vi "TIFFY Cb Crto RGB.vi"(0 "para0":cluster{}, 1 "para4":cluster{}, 2 "para6":cluster{}, 5 "para1":cluster{}, 7 "para2":cluster{}, 9 "para3":cluster{}, 11 "error in (no error)":errorcluster, 12 "para5":cluster{}) -> (3 "para4 out":cluster{}, 4 "para0 out":cluster{}, 6 "para6 out":cluster{}, 8 "function return":u32, 14 "para5 out":cluster{}, 15 "error out":errorcluster)   [LabVIEW 2018]
doc: "LIBTIFF_DLL_IMPEXP void TIFFYCbCrtoRGB(TIFFYCbCrToRGB *, uint32, int32, int32,\n uint32 *, uint32 *, uint32 *);\nextern void TIFFYCbCrtoRGB(TIFFYCbCrToRGB *, uint32, int32, int32,\n uint32 *, uint32 *, uint32 *);"
uses:
  libtiff3.dll
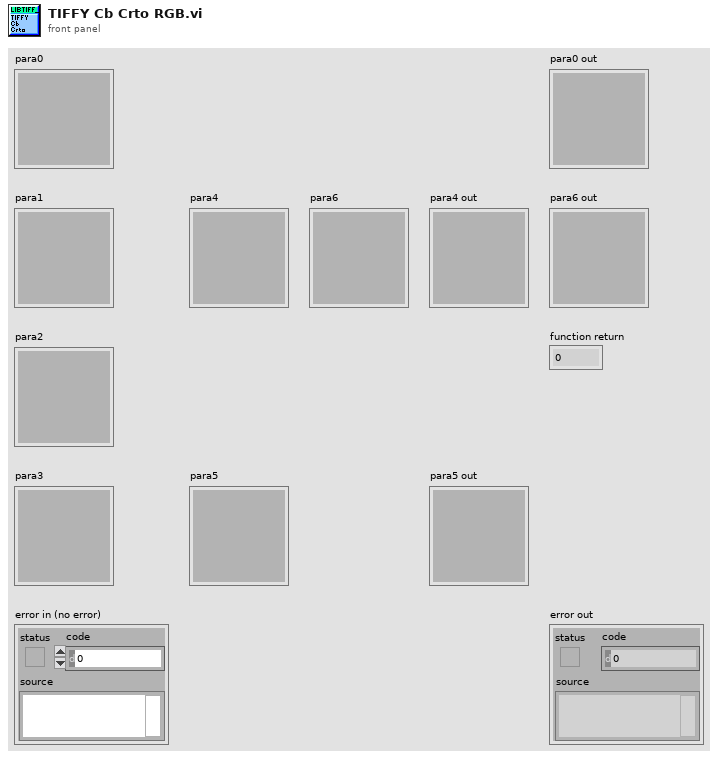
[diagram p1: front panel]
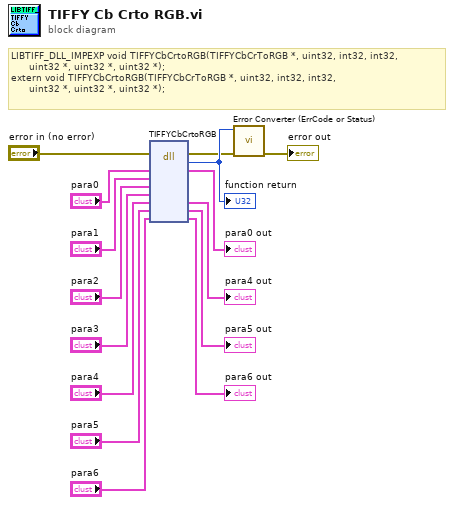
[diagram p0: block diagram]
diagram:
  # "LIBTIFF_DLL_IMPEXP void TIFFYCbCrtoRGB(TIFFYCbCrToRGB *, uint32, int32, int32,\n\t\t\t   uint32 *, uint32 *, uint32 *);\nextern void TIFFYCbCrtoRGB(TIFFYCbCrToRGB *, uint32, int32, int32,\n\t\t\t   uint32 *, uint32 *, uint32 *);"
  n1 = dll-call lib="C:/Users/johan/Downloads/LabVIEW software/LabVIEW software/IX-81 Software/lib/tiff/LibTiffLabview/libtiff3.*" fn="TIFFYCbCrtoRGB"(error in="error in (no error)", "para0"="para0", "para1"="para1", "para2"="para2", "para3"="para3", "para4"="para4", "para5"="para5", "para6"="para6") -> (error out=w2:errorcluster, w15:u32, "para0"=→"para0 out":cluster{}, "para4"=→"para4 out":cluster{}, "para5"=→"para5 out":cluster{}, "para6"=→"para6 out":cluster{})  [unwired: 5 in, 1 out]
  "function return" <- w15
  n2 = call "Error Converter (ErrCode or Status).vi"("error in (no error)"=w2, "error code"=w15) -> ("error out"=→"error out":errorcluster)  [unwired: 9 in]
